vi "Get PowerState.vi"(8 "error in (no error)":errorcluster, 11 "CellPhone in":refnum<class "CellPhone.lvclass">) -> (0 "error out":errorcluster, 2 "PowerState":enum16{"Off", "Sleep", "On"}(ring), 3 "CellPhone out":refnum<class "CellPhone.lvclass">)   [LabVIEW 2009, in "CellPhone.lvclass"]
uses:
  CellPhone.lvclass
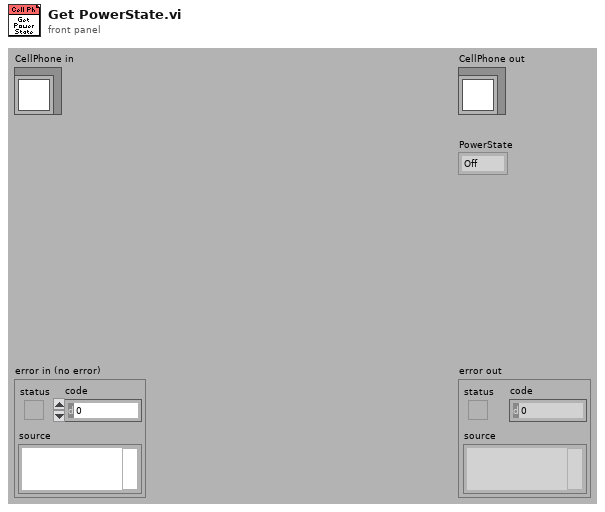
[diagram p1: front panel]
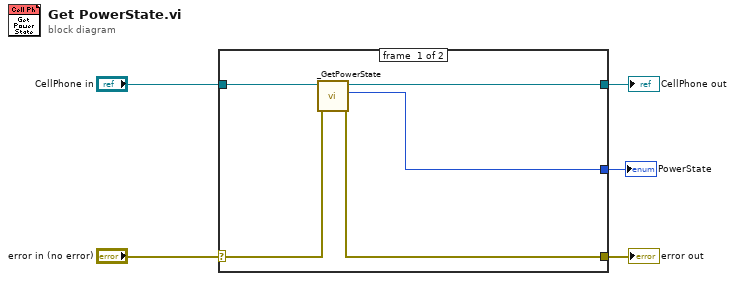
[diagram p0: block diagram]
diagram:
  n1 = case shown="No Error" "error in (no error)" {
    selector: "error in (no error)" -> [w7 w11]
    tunnel: [w6 w11] -> w4
    tunnel: [w9 w12] -> w2
    tunnel: "CellPhone in" -> [w10 w12]
    tunnel: [w8 _] -> w1
    frame #0 {
      n2 = call "_GetPowerState.vi"("error in (no error)"=w7, "CellPhone in"=w10) -> ("error out"=w6:errorcluster, "PowerState"=w8:enum16{"Off", "Sleep", "On"}, "CellPhone out"=w9:refnum<class "CellPhone.lvclass">)  [unwired: 7 in]
    }
    frame #1 {
    }
  }
  "error out" <- w4
  "CellPhone out" <- w2
  "PowerState" <- w1
